vi "#30_MAV_MSG_ATTITUDE_DECODE.vi"(11 "mavlink_payload":u8[](array[numeric])) -> (3 "ATTITUDE":T1)   [LabVIEW 2023]
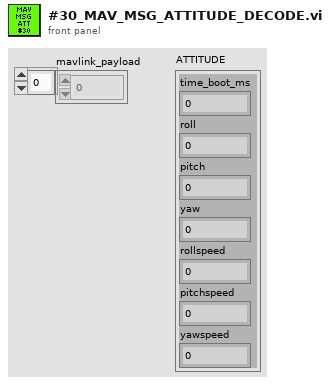
[diagram p1: front panel]
types:
  T1 = cluster{"time_boot_ms":u32, "roll":sgl, "pitch":sgl, "yaw":sgl, "rollspeed":sgl, "pitchspeed":sgl, "yawspeed":sgl}
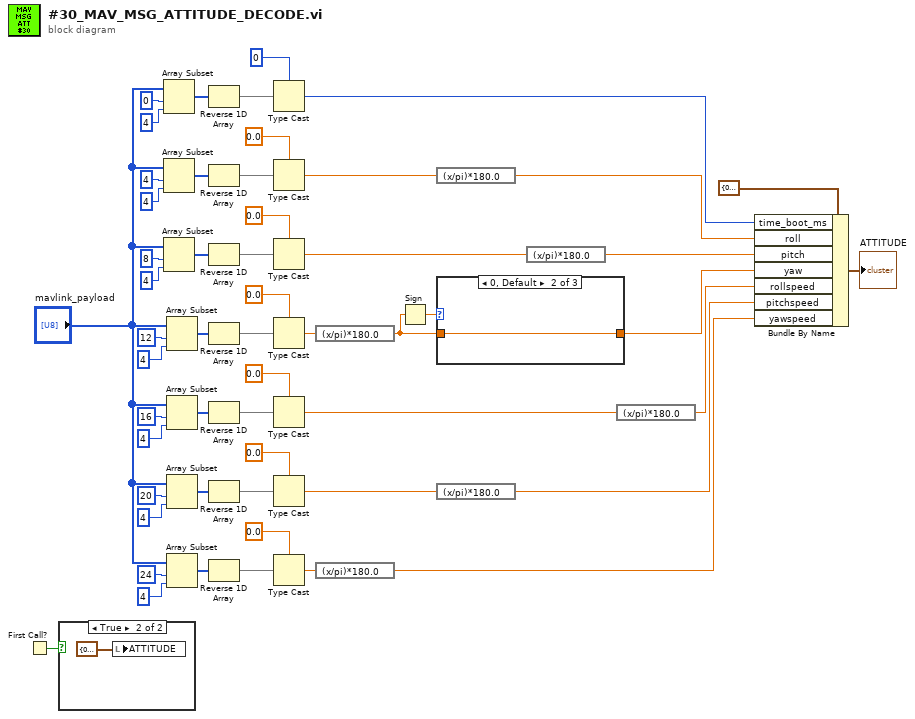
[diagram p0: block diagram]
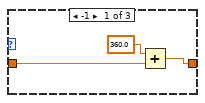
[diagram p3: hidden frame]
diagram:
  n1 = First Call?() -> (First Call?: T/F=w1:bool)
  n2 = case shown="True" w1 {
    frame False {
    }
    frame True {
      n3 = local write "ATTITUDE"(T1 {"time_boot_ms"=0, "roll"=0.0, "pitch"=0.0, "yaw"=0.0, "rollspeed"=0.0, "pitchspeed"=0.0, "yawspeed"=0.0} ("ATTITUDE")) -> ()
    }
  }
  n4 = Array Subset(array="mavlink_payload", index=0, length=4) -> (w54:u8[])
  n5 = Array Subset(array="mavlink_payload", index=4, length=4) -> (w46:u8[])
  n6 = Array Subset(array="mavlink_payload", index=8, length=4) -> (w41:u8[])
  n7 = Array Subset(array="mavlink_payload", index=12, length=4) -> (w36:u8[])
  n8 = Array Subset(array="mavlink_payload", index=16, length=4) -> (w31:u8[])
  n9 = Array Subset(array="mavlink_payload", index=20, length=4) -> (w26:u8[])
  n10 = Array Subset(array="mavlink_payload", index=24, length=4) -> (w21:u8[])
  n11 = Reverse 1D Array(array=w54) -> (reversed array=w53:u8[])
  n12 = Reverse 1D Array(array=w46) -> (reversed array=w45:u8[])
  n13 = Reverse 1D Array(array=w41) -> (reversed array=w40:u8[])
  n14 = Reverse 1D Array(array=w36) -> (reversed array=w35:u8[])
  n15 = Reverse 1D Array(array=w31) -> (reversed array=w30:u8[])
  n16 = Reverse 1D Array(array=w26) -> (reversed array=w25:u8[])
  n17 = Reverse 1D Array(array=w21) -> (reversed array=w20:u8[])
  n18 = Type Cast(type=u32 0 ("single precision float"), x=w53) -> (*(type *) &x=w48:u32)
  n19 = Type Cast(type=sgl 0.0 ("single precision float"), x=w45) -> (*(type *) &x=w13:sgl)
  n20 = Type Cast(type=sgl 0.0 ("single precision float"), x=w40) -> (*(type *) &x=w12:sgl)
  n21 = Type Cast(type=sgl 0.0 ("single precision float"), x=w35) -> (*(type *) &x=w14:sgl)
  n22 = Type Cast(type=sgl 0.0 ("single precision float"), x=w30) -> (*(type *) &x=w9:sgl)
  n23 = Type Cast(type=sgl 0.0 ("single precision float"), x=w25) -> (*(type *) &x=w8:sgl)
  n24 = Type Cast(type=sgl 0.0 ("single precision float"), x=w20) -> (*(type *) &x=w15:sgl)
  n25 = expression code="(x/pi)*180.0" ("radians to degrees")(w14) -> (w3:sgl)
  n26 = expression code="(x/pi)*180.0" ("radians to degrees")(w15) -> (w7:sgl)
  n27 = Sign(1:w3) -> (0:w4:sgl)
  n28 = expression code="(x/pi)*180.0" ("radians to degrees")(w13) -> (w11:sgl)
  n29 = case shown="0, Default" w4 {
    tunnel: w3 -> [w57 w59 w60]
    tunnel: [w56 w59 w60] -> w2
    frame -1 {
      n30 = Add(x=sgl 360.0, y=w57) -> (x+y=w56:sgl)
    }
    frame 0, Default {
    }
    frame 1 {
    }
  }
  n31 = expression code="(x/pi)*180.0" ("radians to degrees")(w8) -> (w5:sgl)
  n32 = expression code="(x/pi)*180.0" ("radians to degrees")(w12) -> (w10:sgl)
  n33 = expression code="(x/pi)*180.0" ("radians to degrees")(w9) -> (w6:sgl)
  n34 = Bundle By Name(cluster=T1 {"time_boot_ms"=0, "roll"=0.0, "pitch"=0.0, "yaw"=0.0, "rollspeed"=0.0, "pitchspeed"=0.0, "yawspeed"=0.0} ("ATTITUDE"), "time_boot_ms"=w48, "roll"=w11, "pitch"=w10, "yaw"=w2, "rollspeed"=w6, "pitchspeed"=w5, "yawspeed"=w7) -> (→"ATTITUDE":T1)
